vi "AOTF-4ch-Trigger.vi"() -> ()   [LabVIEW 2011]
doc: "I. Description:\nThis example demonstrates how to generate a continuous digital pulse train from a Counter Output Channel started by an external digital trigger. The Frequency, Duty Cycle, and Idle State are all configurable. \n\nThis example shows how to configure the pulse in terms of Frequency/Duty Cycle, but can easily be modified to generate a pulse in terms of Time or Ticks.\n\nII. Instructions for Running:\n1. Select the Physical Channel which corresponds to the counter you want to output your signal to on the DAQ device.\n2. Enter the Frequency and Duty Cycle to define the pulse parameters. You can also change the Idle State to set the state the line will remain in after the generation is stopped. Additionally, you can set the Initial Delay (in seconds) which will delay the beginning of the pulse train from the start call; this is currently wired to 0.0 on the block diagram. \n3. Setup the Trigger Parameters. In this example the VI is expecting a Rising Edge Digital Trigger on PFI9. \n\nIII. Block Diagram Steps:\n1. Create a Counter Output channel to produce a Pulse in terms of Frequency. If the Idle State of the pulse is set to low the first transition of the generated signal is from low to high.\n2. Use the DAQmx Trigger VI to configure a trigger to start on a digital edge.\n2. Use the DAQmx Timing VI (Implicit) to configure the duration of the pulse generation.\n3. Call the Start VI to arm the counter and begin the pulse train generation.\n4. Loop continuously until the user presses the Stop button. Check for errors every 100 ms using the Is Task Done? VI\n5. Call the Clear Task VI to clear the Task.\n\nIV. I/O Connections Overview:\nThe counter will output the pulse train on the output terminal of the counter specified in the Physical Channel I/O control. \n\nIn this example the output will be sent to the default output terminal on ctr0.\n\nFor more information on the default counter input and output terminals for your device, open the NI-DAQmx Help, and refer to Counter Signal Connections found under the Device Considerations book in the table of contents."
uses:
  <vilib>/Utility/error.llb/DialogType.ctl
  <vilib>/DAQmx/create/channels.llb/DAQmx Create Channel (CO-Pulse Generation-Frequency).vi
  <vilib>/DAQmx/configure/trigger.llb/DAQmx Start Trigger (Digital Edge).vi
  <vilib>/DAQmx/configure/timing.llb/DAQmx Timing (Implicit).vi
panel:
  in  "Duty Cycle 4":dbl=0.5 caption="Duty Cycle" format="%0.2f"
  in  "Duty Cycle 3":dbl=0.5 caption="Duty Cycle" format="%0.2f"
  in  "Duty Cycle 2":dbl=0.5 caption="Duty Cycle" format="%0.2f"
  in  "Counter 4":tag="Dev1/ctr0"
  in  "Counter 3":tag="Dev1/ctr0"
  in  "Channel 4":bool
  in  "Channel 3":bool
  in  "Channel 2":bool
  in  "Channel 1":bool
  in  "Idle State 2":i32(ring)=10214 caption="Idle State" items=["High"=10192, "Low"=10214]
  in  "Counter 1":tag="Dev1/ctr0"
  in  "Trigger Edge":i32(ring)=10280 items=["Rising"=10280, "Falling"=10171]
  in  "Trigger Source":tag="/Dev1/PFI9"
  in  "Duty Cycle  1":dbl=0.5 caption="Duty Cycle" format="%0.2f"
  in  "Frequency":dbl=1.0 caption="Frequency (kHz)" format="%0.2f"
  in  "Idle State":i32(ring)=10214 items=["High"=10192, "Low"=10214]
  in  "Counter 2":tag="Dev1/ctr0"
  in  "Stop":bool caption="stop"
  # "Channel Parameters"
  # "Trigger Parameters"
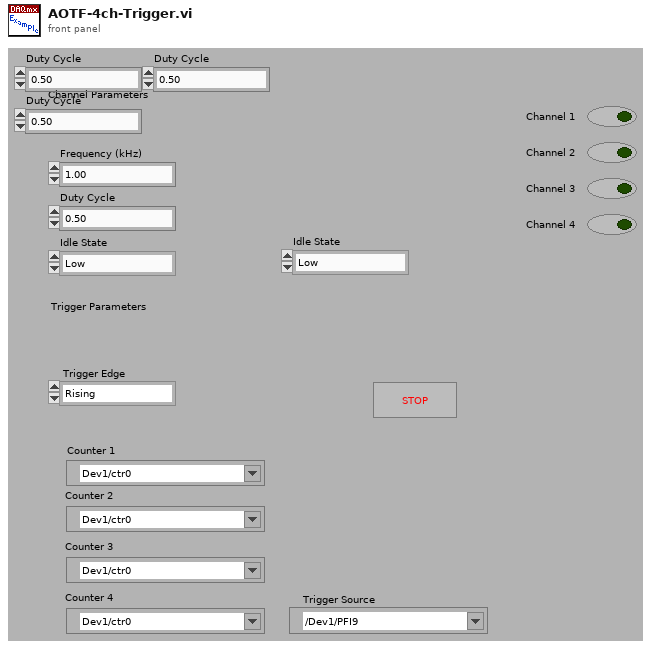
[diagram p1: front panel]
types:
  T1 = typedef "DialogType.ctl" = u16
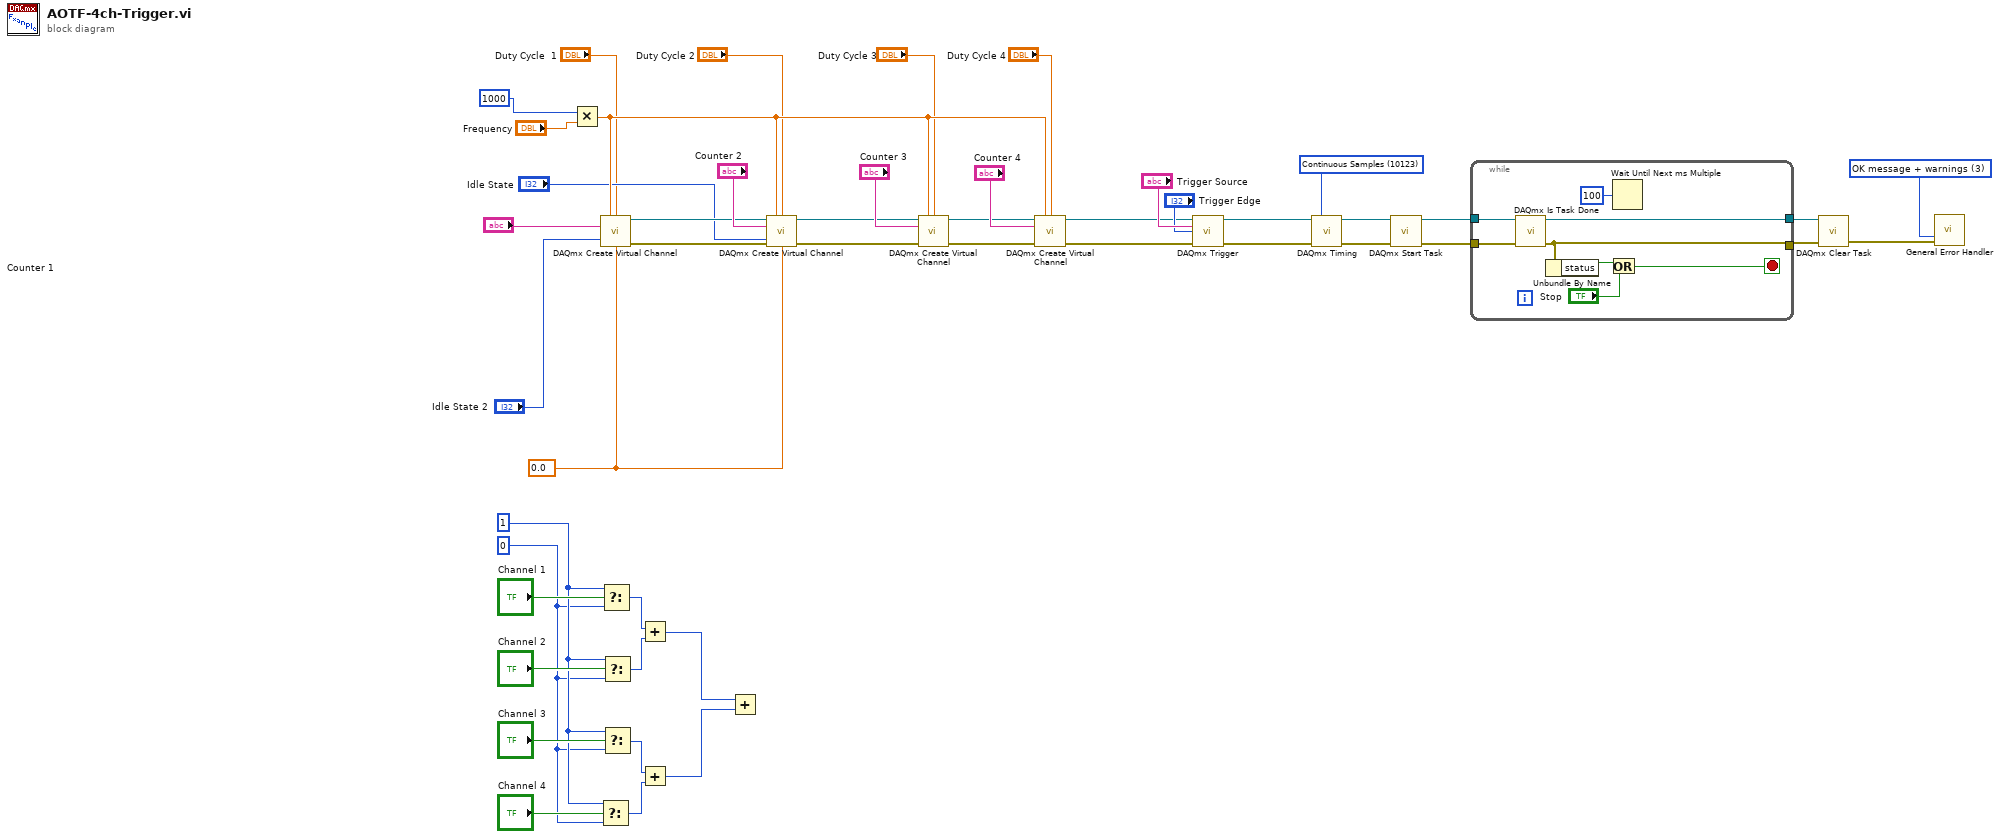
[diagram p0: block diagram]
diagram:
  w19 = 1
  w18 = 0
  w37 = T1 3 items=["no dialog", "OK message", "continue or stop message", "OK message + warnings", "continue/stop + warnings"] ("type of dialog (OK msg:1)")
  w34 = 0.0 ("initial delay")
  w43 = 10123 items=["Finite Samples"=10178, "Continuous Samples"=10123] ("sample mode")
  n1 = Multiply(x=1000, y="Frequency") -> (x*y=w6:dbl)
  n2 = call-poly <vilib>:"DAQmx Create Virtual Channel.vi"("frequency"=w6, "duty cycle"="Duty Cycle  1", "counter"="Counter 1", "idle state"="Idle State 2", "initial delay"=w34) -> ("task out"=w33:refnum<k21>, "error out"=w35:errorcluster)  [unwired: 9 in]
  n3 = Select(t=w19, s="Channel 4", f=w18) -> (s? t:f=w20:i32)
  n4 = Select(t=w19, s="Channel 1", f=w18) -> (s? t:f=w26:i32)
  n5 = Select(t=w19, s="Channel 2", f=w18) -> (s? t:f=w22:i32)
  n6 = Select(t=w19, s="Channel 3", f=w18) -> (s? t:f=w21:i32)
  n7 = Add(x=w26, y=w22) -> (x+y=w28:i32)
  n8 = Add(x=w21, y=w20) -> (x+y=w29:i32)
  n9 = Add(x=w28, y=w29) -> ()  [unwired: 1 out]
  n10 = call-poly <vilib>:"DAQmx Create Virtual Channel.vi"("task in"=w33, "frequency"=w6, "duty cycle"="Duty Cycle 2", "counter"="Counter 2", "error in"=w35, "idle state"="Idle State", "initial delay"=w34) -> ("task out"=w11:refnum<k21>, "error out"=w14:errorcluster)  [unwired: 7 in]
  n11 = call-poly <vilib>:"DAQmx Create Virtual Channel.vi"("task in"=w11, "frequency"=w6, "duty cycle"="Duty Cycle 3", "counter"="Counter 3", "error in"=w14) -> ("task out"=w12:refnum<k21>, "error out"=w15:errorcluster)  [unwired: 9 in]
  n12 = call-poly <vilib>:"DAQmx Create Virtual Channel.vi"("task in"=w12, "frequency"=w6, "duty cycle"="Duty Cycle 4", "counter"="Counter 4", "error in"=w15) -> ("task out"=w10:refnum<k21>, "error out"=w13:errorcluster)  [unwired: 9 in]
  n13 = call-poly <vilib>:"DAQmx Trigger.vi"("task/channels in"=w10, "source"="Trigger Source", "edge"="Trigger Edge", "error in"=w13) -> ("task out"=w41:refnum<k21>, "error out"=w40:errorcluster)  [unwired: 10 in]
  n14 = call-poly <vilib>:"DAQmx Timing.vi"("task/channels in"=w41, "sample mode"=w43, "error in"=w40) -> ("task out"=w44:refnum<k21>, "error out"=w45:errorcluster)  [unwired: 11 in]
  n15 = call <vilib>:"DAQmx Start Task.vi"("task/channels in"=w44, "error in"=w45) -> ("task out"=w47:refnum<k21>, "error out"=w9:errorcluster)  [unwired: 12 in]
  n16 = while {
    tunnel: w9 -> [w54]
    tunnel: w47 -> [w55]
    tunnel: [w53] -> w46
    tunnel: [w52] -> w8
    stop <- w50 stop-if-true
    n17 = call <vilib>:"DAQmx Is Task Done.vi"("task/channels in"=w55, "error in"=w54) -> ("task out"=w53:refnum<k21>, "error out"=w52:errorcluster)  [unwired: 11 in, 1 out]
    n18 = Unbundle By Name(w52) -> ("status"=w49:bool)
    n19 = Or(x=w49, y="Stop") -> (x .or. y?=w50:bool)
    n20 = Wait Until Next ms Multiple(millisecond multiple=u32 100) -> ()  [unwired: 1 out]
  }
  n21 = call <vilib>:"DAQmx Clear Task.vi"("task in"=w46, "error in"=w8) -> ("error out"=w7:errorcluster)  [unwired: 13 in]
  n22 = call <vilib>:"General Error Handler.vi"("type of dialog (OK msg:1)"=w37, "error in (no error)"=w7) -> ()  [unwired: 9 in, 5 out]
